vi "SP Print Test Panel.vi"(7 "Plot References":refnum<vi>[](array[refnum]), 8 "error in (no error)":errorcluster, 11 "VI Reference":refnum<vi>) -> (0 "error out":errorcluster)   [LabVIEW 2011]
uses:
  <vilib>/Utility/miscctls.llb/LVPrintingMarginsTypeDef.ctl
  TypeDefs/SP Plot Cluster Object.ctl
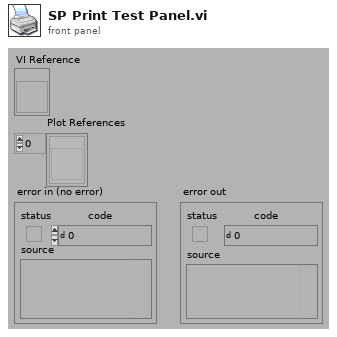
[diagram p1: front panel]
types:
  T1 = typedef "SP Plot Cluster Object.ctl" = enum16{"Plot", "CH Reference", "CH Label", "Start Label", "Stop Label", "Units Label", "Selected?", "CH Markers"}
  T2 = typedef "LVPrintingMarginsTypeDef.ctl" = cluster{"Top":sgl, "Left":sgl, "Bottom":sgl, "Right":sgl, "Measurement System":enum8{"Inches", "cm"}}
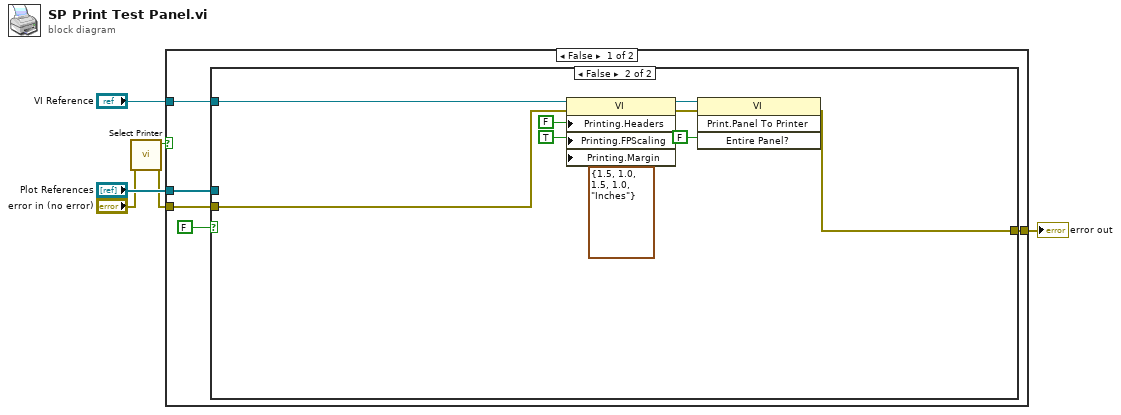
[diagram p0: block diagram]
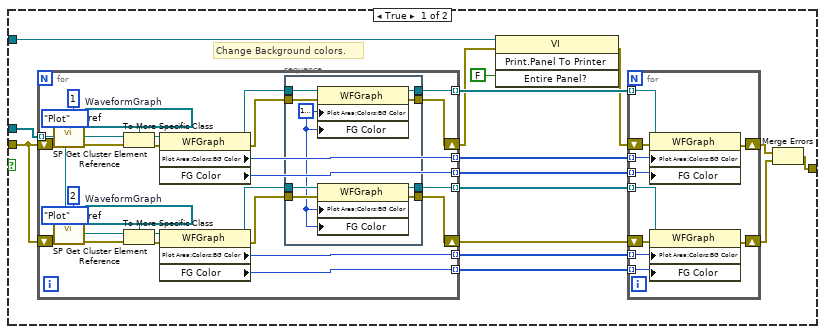
[diagram p2: hidden frame]
diagram:
  n1 = call "Select Printer.vi"("error in (no error)"="error in (no error)") -> ("error out"=w2:errorcluster, "Canceled?"=w1:bool)  [unwired: 9 out]
  n2 = case shown="False" w1 {
    tunnel: "VI Reference" -> [w11 _]
    tunnel: "Plot References" -> [w10 _]
    tunnel: [w9 w83] -> w4
    tunnel: w2 -> [w8 w83]
    frame False {
      n3 = case shown="False" FALSE {
        tunnel: w11 -> [w26 w78]
        tunnel: w10 -> [w25 _]
        tunnel: [w22 w81] -> w9
        tunnel: w8 -> [w12 w80]
        frame True {
          # "Change Background colors."
          n4 = for {
            tunnel: w25 -> [w38] mode=indexing
            shift-right: [w55] -> w23
            shift-left: w12 -> [w56]
            tunnel: [w54] -> w24 mode=indexing
            tunnel: [w53] -> w21 mode=indexing
            tunnel: [w52] -> w20 mode=indexing
            shift-right: [w48] -> w16
            shift-left: w12 -> [w47]
            tunnel: [w49] -> w17 mode=indexing
            tunnel: [w50] -> w18 mode=indexing
            tunnel: [w51] -> w19 mode=indexing
            w45 = refnum<vi> refnum  # WaveformGraph
            w58 = refnum<vi> refnum  # WaveformGraph
            n5 = call "SP Get Cluster Element Reference.vi"("Channel"=1, "Element"=SP_Plot_Cluster_Object."Plot", "Plot Reference"=w38) -> ("Element Reference"=w43:refnum<vi>)  [unwired: 6 out]
            n6 = call "SP Get Cluster Element Reference.vi"("Channel"=2, "Element"=SP_Plot_Cluster_Object."Plot", "Plot Reference"=w38) -> ("Element Reference"=w60:refnum<vi>)  [unwired: 6 out]
            n7 = To More Specific Class(target class=w45, reference=w43, error in=w47) -> (specific class reference=w42:refnum<vi>, error out=w39:errorcluster)
            n8 = To More Specific Class(target class=w58, reference=w60, error in=w56) -> (specific class reference=w61:refnum<vi>, error out=w64:errorcluster)
            n9 = property on="Property Node" class="WFGraph"(reference=w42, error in=w39) -> (reference out=w41:refnum<vi>, error out=w40:errorcluster, "Plot Area:Colors:BG Color"=w50:u32, "FG Color"=w51:u32)
            n10 = property on="Property Node" class="WFGraph"(reference=w61, error in=w64) -> (reference out=w62:refnum<vi>, error out=w63:errorcluster, "Plot Area:Colors:BG Color"=w53:u32, "FG Color"=w52:u32)
            n11 = stacked-sequence {
              tunnel: w63 -> [w73]
              tunnel: w62 -> [w72]
              tunnel: [w71] -> w55
              tunnel: [w70] -> w54
              tunnel: [w69] -> w49
              tunnel: [w68] -> w48
              tunnel: w41 -> [w67]
              tunnel: w40 -> [w66]
              frame #0 {
                w65 = u32 16777222 ("Color")
                n12 = property on="Property Node" class="WFGraph"(reference=w67, error in=w66, "Plot Area:Colors:BG Color"=w65, "FG Color"=w65) -> (reference out=w69:refnum<vi>, error out=w68:errorcluster)
                n13 = property on="Property Node" class="WFGraph"(reference=w72, error in=w73, "Plot Area:Colors:BG Color"=w65, "FG Color"=w65) -> (reference out=w70:refnum<vi>, error out=w71:errorcluster)
              }
            }
          }
          n14 = invoke class="VI" method="Print.Panel To Printer"(reference=w26, error in=w16, "Entire Panel?"=FALSE) -> (error out=w15:errorcluster)  [unwired: 1 in, 3 out]
          n15 = for {
            tunnel: w24 -> [w37] mode=indexing
            shift-right: [w35] -> w14
            shift-left: w23 -> [w36]
            tunnel: w21 -> [w34] mode=indexing
            tunnel: w20 -> [w33] mode=indexing
            tunnel: w17 -> [w28] mode=indexing
            shift-right: [w30] -> w13
            shift-left: w15 -> [w29]
            tunnel: w18 -> [w31] mode=indexing
            tunnel: w19 -> [w32] mode=indexing
            n16 = property on="Property Node" class="WFGraph"(reference=w28, error in=w29, "Plot Area:Colors:BG Color"=w31, "FG Color"=w32) -> (error out=w30:errorcluster)  [unwired: 1 out]
            n17 = property on="Property Node" class="WFGraph"(reference=w37, error in=w36, "Plot Area:Colors:BG Color"=w34, "FG Color"=w33) -> (error out=w35:errorcluster)  [unwired: 1 out]
          }
          n18 = Merge Errors(w13, w14) -> (w22:errorcluster)
        }
        frame False {
          n19 = property class="VI"(reference=w78, error in=w80, "Printing.Headers"=FALSE ("Printing:Page Headers?"), "Printing.FPScaling"=TRUE ("Printing:Front Panel Scaling?"), "Printing.Margin"=T2 {"Top"=1.5, "Left"=1.0, "Bottom"=1.5, "Right"=1.0, "Measurement System"=enum."Inches"} ("Printing:Margins")) -> (reference out=w77:refnum<vi>, error out=w79:errorcluster)
          n20 = invoke class="VI" method="Print.Panel To Printer"(reference=w77, error in=w79, "Entire Panel?"=FALSE) -> (error out=w81:errorcluster)  [unwired: 1 in, 3 out]
        }
      }
    }
    frame True {
    }
  }
  "error out" <- w4
